vi "RichToFlatni_measurementlink_sessionmanagement_v1_GetSessionsResponse.vi"(5 "OutputClusterType":T1, 11 "InputCluster":T8) -> (3 "OutputCluster":T1)   [LabVIEW 2021, in "ni.measurementlink.sessionmanagement.v1.api.lvlib"]
uses:
  ni.measurementlink.sessionmanagement.v1.api.lvlib
  ni_measurementlink_sessionmanagement_v1_MultiplexerSessionInformation_AnnotationsEntry_Flat.ctl
  nidevice_grpc_Session_Flat.ctl
  ni_measurementlink_sessionmanagement_v1_MultiplexerSessionInformation_Flat.ctl
  ni_measurementlink_sessionmanagement_v1_SessionInformation_AnnotationsEntry_Flat.ctl
  ni_measurementlink_sessionmanagement_v1_ChannelMapping_Flat.ctl
  ni_measurementlink_sessionmanagement_v1_SessionInformation_Flat.ctl
  ni_measurementlink_sessionmanagement_v1_GetSessionsResponse_Flat.ctl
  ni_measurementlink_sessionmanagement_v1_MultiplexerSessionInformation_AnnotationsEntry.ctl
  nidevice_grpc_Session.ctl
  ni_measurementlink_sessionmanagement_v1_MultiplexerSessionInformation.ctl
  ni_measurementlink_sessionmanagement_v1_SessionInformation_AnnotationsEntry.ctl
  ni_measurementlink_sessionmanagement_v1_ChannelMapping.ctl
  ni_measurementlink_sessionmanagement_v1_SessionInformation.ctl
  ni_measurementlink_sessionmanagement_v1_GetSessionsResponse.ctl
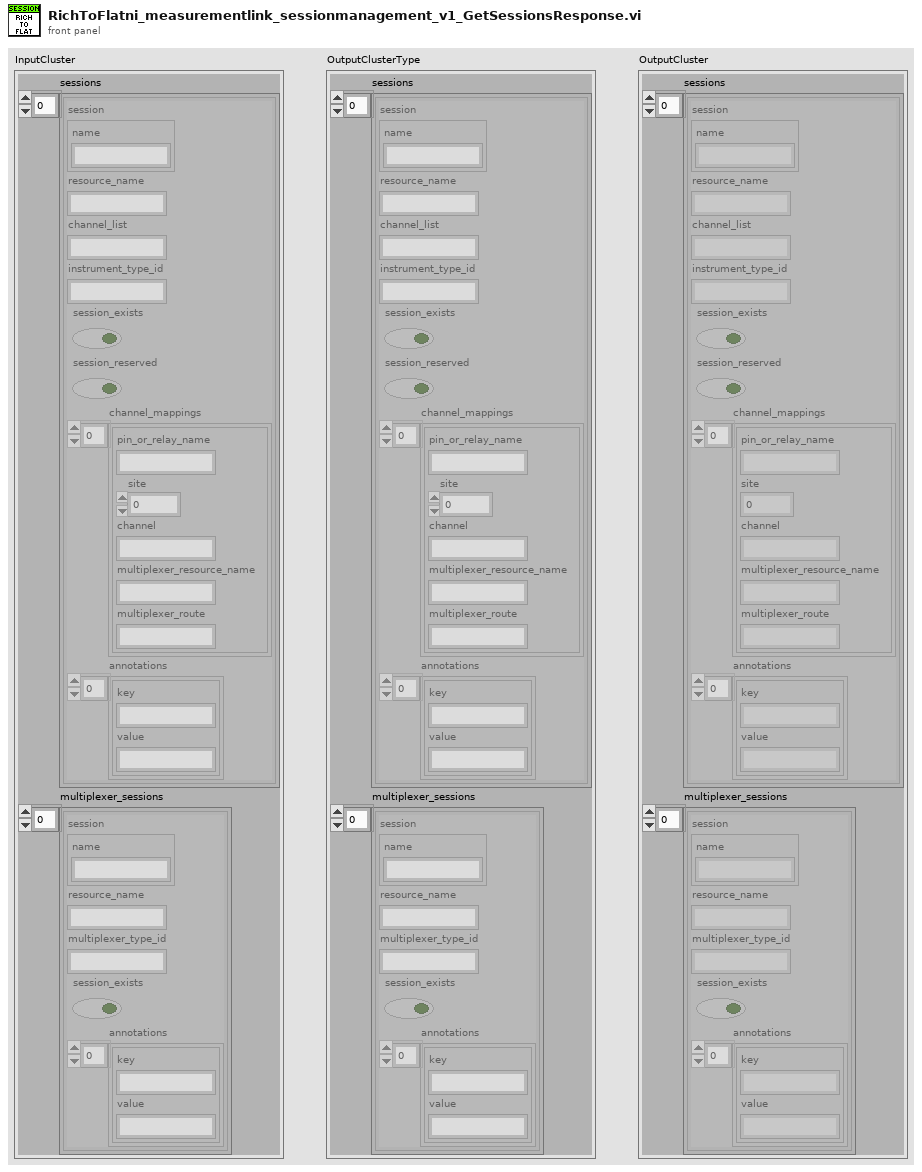
[diagram p1: front panel]
types:
  T1 = typedef "ni.measurementlink.sessionmanagement.v1.api.lvlib/ni_measurementlink_sessionmanagement_v1_GetSessionsResponse_Flat.ctl" = cluster{"sessions":T2[], "multiplexer_sessions":T6[]}
  T2 = typedef "ni.measurementlink.sessionmanagement.v1.api.lvlib/ni_measurementlink_sessionmanagement_v1_SessionInformation_Flat.ctl" = cluster{"session":T3, "resource_name":string, "channel_list":string, "instrument_type_id":string, "session_exists":bool, "session_reserved":bool, "channel_mappings":T4[], "annotations":T5[]}
  T3 = typedef "ni.measurementlink.sessionmanagement.v1.api.lvlib/nidevice_grpc_Session_Flat.ctl" = cluster{"name":string}
  T4 = typedef "ni.measurementlink.sessionmanagement.v1.api.lvlib/ni_measurementlink_sessionmanagement_v1_ChannelMapping_Flat.ctl" = cluster{"pin_or_relay_name":string, "site":i32, "channel":string, "multiplexer_resource_name":string, "multiplexer_route":string}
  T5 = typedef "ni.measurementlink.sessionmanagement.v1.api.lvlib/ni_measurementlink_sessionmanagement_v1_SessionInformation_AnnotationsEntry_Flat.ctl" = cluster{"key":string, "value":string}
  T6 = typedef "ni.measurementlink.sessionmanagement.v1.api.lvlib/ni_measurementlink_sessionmanagement_v1_MultiplexerSessionInformation_Flat.ctl" = cluster{"session":T3, "resource_name":string, "multiplexer_type_id":string, "session_exists":bool, "annotations":T7[]}
  T7 = typedef "ni.measurementlink.sessionmanagement.v1.api.lvlib/ni_measurementlink_sessionmanagement_v1_MultiplexerSessionInformation_AnnotationsEntry_Flat.ctl" = cluster{"key":string, "value":string}
  T8 = typedef "ni.measurementlink.sessionmanagement.v1.api.lvlib/ni_measurementlink_sessionmanagement_v1_GetSessionsResponse.ctl" = cluster{"sessions":T9[], "multiplexer_sessions":T13[]}
  T9 = typedef "ni.measurementlink.sessionmanagement.v1.api.lvlib/ni_measurementlink_sessionmanagement_v1_SessionInformation.ctl" = cluster{"session":T10, "resource_name":string, "channel_list":string, "instrument_type_id":string, "session_exists":bool, "session_reserved":bool, "channel_mappings":T11[], "annotations":T12[]}
  T10 = typedef "ni.measurementlink.sessionmanagement.v1.api.lvlib/nidevice_grpc_Session.ctl" = cluster{"name":string}
  T11 = typedef "ni.measurementlink.sessionmanagement.v1.api.lvlib/ni_measurementlink_sessionmanagement_v1_ChannelMapping.ctl" = cluster{"pin_or_relay_name":string, "site":i32, "channel":string, "multiplexer_resource_name":string, "multiplexer_route":string}
  T12 = typedef "ni.measurementlink.sessionmanagement.v1.api.lvlib/ni_measurementlink_sessionmanagement_v1_SessionInformation_AnnotationsEntry.ctl" = cluster{"key":string, "value":string}
  T13 = typedef "ni.measurementlink.sessionmanagement.v1.api.lvlib/ni_measurementlink_sessionmanagement_v1_MultiplexerSessionInformation.ctl" = cluster{"session":T10, "resource_name":string, "multiplexer_type_id":string, "session_exists":bool, "annotations":T14[]}
  T14 = typedef "ni.measurementlink.sessionmanagement.v1.api.lvlib/ni_measurementlink_sessionmanagement_v1_MultiplexerSessionInformation_AnnotationsEntry.ctl" = cluster{"key":string, "value":string}
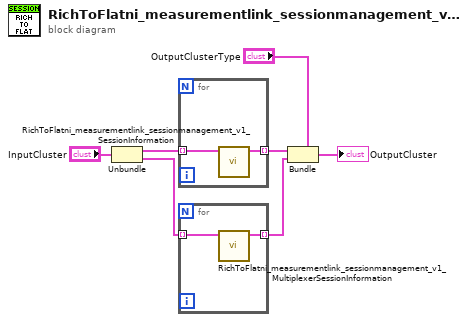
[diagram p0: block diagram]
diagram:
  n1 = Unbundle "Unbundle"("InputCluster") -> ("sessions"=w4:T9[], "multiplexer_sessions"=w2:T13[])
  n2 = for {
    tunnel: w4 -> [w9] mode=indexing
    tunnel: [w8] -> w3 mode=indexing
    n3 = call "RichToFlatni_measurementlink_sessionmanagement_v1_SessionInformation.vi"("InputCluster"=w9) -> ("OutputCluster"=w8:T2)  [unwired: 10 in]
  }
  n4 = for {
    tunnel: w2 -> [w11] mode=indexing
    tunnel: [w10] -> w1 mode=indexing
    n5 = call "RichToFlatni_measurementlink_sessionmanagement_v1_MultiplexerSessionInformation.vi"("InputCluster"=w11) -> ("OutputCluster"=w10:T6)  [unwired: 10 in]
  }
  n6 = Bundle "Bundle"(cluster="OutputClusterType", "sessions"=w3, "multiplexer_sessions"=w1) -> (→"OutputCluster":T1)
